vi "system get Input Voltage LV.vi"(8 "error in (no error)":errorcluster, 10 "result":cluster{"value":i32, "error":i32}, 11 "id":i32) -> (0 "error out":errorcluster, 2 "result out":cluster{"value":i32, "error":i32}, 3 "id out":i32)   [LabVIEW 2015, in "BrainStem4LabView.lvlib"]
doc: "__declspec(dllexport) void __stdcall system_getInputVoltage_LV(int* id, struct Result* result);"
uses:
  BrainStem4LabView.lvlib
  LabViewTesting.dll
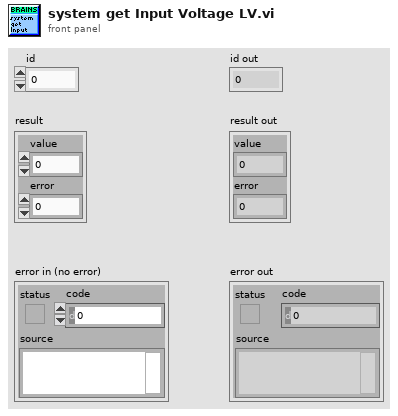
[diagram p1: front panel]
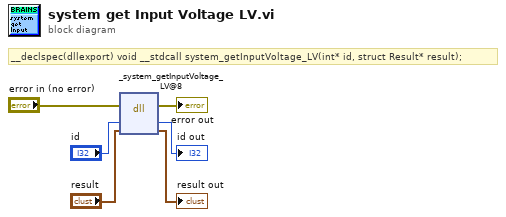
[diagram p0: block diagram]
diagram:
  # "__declspec(dllexport) void __stdcall system_getInputVoltage_LV(int* id, struct Result* result);"
  n1 = dll-call lib="C:/Users/Acroname_User/development/acroname/software/acroname/aSource/LabVIEW/LabView_BS_Project/BrainStem_DLL_Import/LabViewTesting.*" fn="_system_getInputVoltage_LV@8"(error in="error in (no error)", "id"="id", "result"="result") -> (error out=→"error out":errorcluster, "id"=→"id out":i32, "result"=→"result out":cluster{"value":i32, "error":i32})  [unwired: 3 in, 1 out]
